vi "send_error.vi"(7 "JSON Tree In (JSON Object)":variant, 8 "error in":errorcluster, 9 "timeout ms":i32, 11 "connection ID":refnum<k5>) -> (0 "error out":errorcluster, 1 "bytes":string, 2 "#bytes written":i32, 3 "connection ID out":refnum<k5>)   [LabVIEW 2010]
uses:
  i3-json-1.0.0-10/JSON Generation/Create Value Files/Create Value - Object.vi
  i3-json-1.0.0-10/JSON Generation/Add Object Parameter Files/Add Object Parameter - String.vi
  i3-json-1.0.0-10/JSON Generation/Add Object Parameter Files/Add Object Parameter - Boolean.vi
  i3-json-1.0.0-10/JSON Generation/Add Object Parameter Files/Add Object Parameter - 1D Array String.vi
  i3-json-1.0.0-10/JSON Generation/Add Object Parameter Files/Add Object Parameter - Null.vi
  i3-json-1.0.0-10/JSON Parsing/Get Object Parameter Files/Get Object Parameter - String.vi
  i3-json-1.0.0-10/i3-json.lvlib
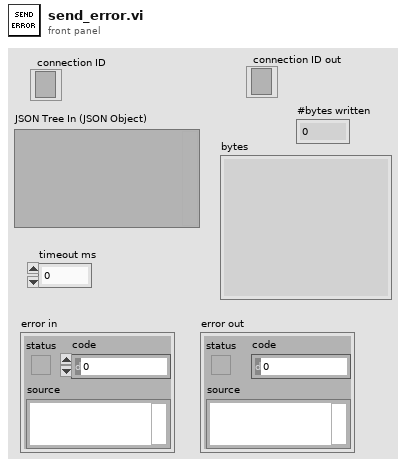
[diagram p1: front panel]
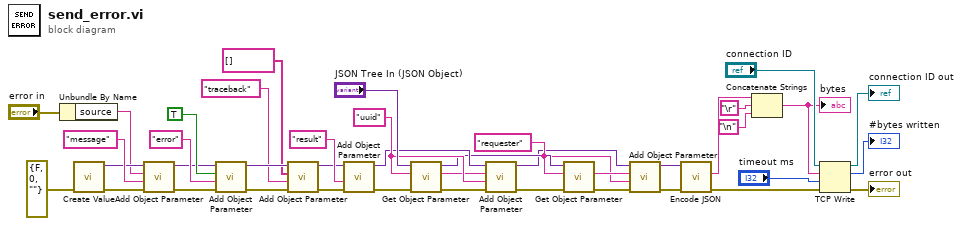
[diagram p0: block diagram]
diagram:
  w27 = "uuid" ("name")
  w20 = "requester" ("name")
  n1 = Unbundle By Name("error in") -> ("source"=w12:string)
  n2 = call-poly "Create Value.vi"("error in (no error)"=errorcluster {"status"=FALSE, "code"=0, "source"=""}) -> ("error out"=w13:errorcluster, "JSON Tree"=w14:variant)  [unwired: 9 in]
  n3 = call-poly "Add Object Parameter.vi"("error in (no error)"=w13, "Name"="message", "String"=w12, "JSON Tree in (JSON Object)"=w14) -> ("error out"=w10:errorcluster, "JSON Tree out (JSON Object)"=w11:variant)  [unwired: 6 in]
  n4 = call-poly "Add Object Parameter.vi"("error in (no error)"=w10, "Name"="error", "Boolean"=TRUE, "JSON Tree in (JSON Object)"=w11) -> ("error out"=w8:errorcluster, "JSON Tree out (JSON Object)"=w9:variant)  [unwired: 6 in]
  n5 = call-poly "Add Object Parameter.vi"("error in (no error)"=w8, "Name"="traceback", "1D String"=string[] [], "JSON Tree in (JSON Object)"=w9) -> ("error out"=w5:errorcluster, "JSON Tree out (JSON Object)"=w6:variant)  [unwired: 6 in]
  n6 = call-poly "Add Object Parameter.vi"("error in (no error)"=w5, "Name"="result" ("Default Value if JSON Null"), "JSON Tree in (JSON Object)"=w6) -> ("error out"=w29:errorcluster, "JSON Tree out (JSON Object)"=w25:variant)  [unwired: 7 in]
  n7 = call-poly "Get Object Parameter.vi"("error in (no error)"=w29, "Parameter Name"=w27, "JSON Tree In (JSON Object)"="JSON Tree In (JSON Object)") -> ("error out"=w28:errorcluster, "String Value"=w26:string, "JSON Tree Out Passthrough"=w21:variant)  [unwired: 5 in, 1 out]
  n8 = call-poly "Add Object Parameter.vi"("error in (no error)"=w28, "Name"=w27, "String"=w26, "JSON Tree in (JSON Object)"=w25) -> ("error out"=w22:errorcluster, "JSON Tree out (JSON Object)"=w19:variant)  [unwired: 6 in]
  n9 = call-poly "Get Object Parameter.vi"("error in (no error)"=w22, "Parameter Name"=w20, "JSON Tree In (JSON Object)"=w21) -> ("error out"=w23:errorcluster, "String Value"=w24:string)  [unwired: 5 in, 2 out]
  n10 = call-poly "Add Object Parameter.vi"("error in (no error)"=w23, "Name"=w20, "String"=w24, "JSON Tree in (JSON Object)"=w19) -> ("error out"=w3:errorcluster, "JSON Tree out (JSON Object)"=w4:variant)  [unwired: 6 in]
  n11 = call "Encode JSON.vi"("error in (no error)"=w3, "JSON Tree"=w4) -> ("error out"=w2:errorcluster, "String"=w35:string)  [unwired: 4 in]
  n12 = Concatenate Strings(w35, "\r", "\n") -> (w32:string)
  "bytes" <- w32
  n13 = TCP Write(connection ID="connection ID", data in=w32, error in (no error)=w2, 9:"timeout ms") -> (connection ID out=→"connection ID out":refnum<k5>, bytes written=→"#bytes written":i32, error out=→"error out":errorcluster)
